vi "Get ComponentPath.vi"(8 "error in (no error)":errorcluster, 10 "BrowerComponentID(\"\")":string, 11 "BrowerTree in":refnum<class "BrowerTree.lvclass">) -> (0 "error out":errorcluster, 2 "Navigate Tree:Get Paths":string[](array[string]), 3 "BrowerTree out":refnum<class "BrowerTree.lvclass">)   [LabVIEW 2015, in "BrowerTree.lvclass"]
uses:
  BrowerTree.lvclass
  BrowerTree.lvclass/BrowerTree.ctl
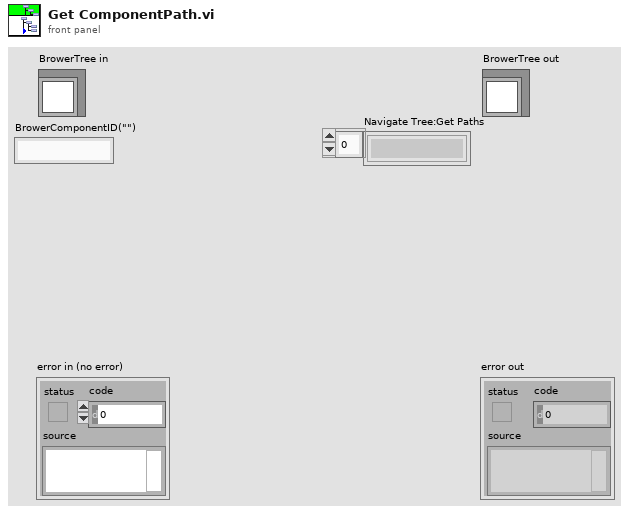
[diagram p1: front panel]
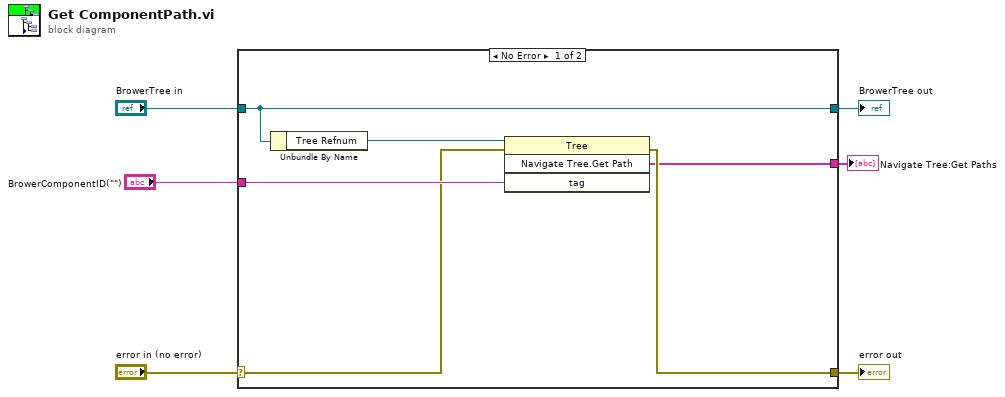
[diagram p0: block diagram]
diagram:
  n1 = case shown="No Error" "error in (no error)" {
    selector: "error in (no error)" -> [w9 w14]
    tunnel: [w8 w14] -> w5
    tunnel: [w12 w13] -> w3
    tunnel: "BrowerTree in" -> [w12 w13]
    tunnel: "BrowerComponentID(\"\")" -> [w10 _]
    tunnel: [w7 _] -> w1
    frame No Error {
      n2 = Unbundle By Name(w12) -> ("Tree Refnum"=w11:refnum<vi>)
      n3 = invoke class="Tree" method="Navigate Tree.Get Path"(reference=w11, error in=w9, "tag"=w10) -> (error out=w8:errorcluster, "Navigate Tree:Get Path"=w7:string[])  [unwired: 1 in, 2 out]
    }
    frame Error {
    }
  }
  "error out" <- w5
  "BrowerTree out" <- w3
  "Navigate Tree:Get Paths" <- w1
